vi "Settings Dialog.vi"(8 "error in (no error)":errorcluster, 11 "Settings in":T5={"Acquisition Settings"={"AI"={"task name"="", "task_ref"="", "physical channels"="Dev1/ai0:7", "channels config"={"input terminal configuration"=0, "minimum value"=-5.0, "maximum value"=5.0}, "rate"=1000.0}, "conversions"={"ai0"={"a"=0.0, "b"=0.0}, "ai1"={"a"=0.0, "b"=0.0}, "ai2"={"a"=0.0, "b"=0.0}, "ai3"={"a"=0.0, "b"=0.0}, "ai4"={"a"=0.0, "b"=0.0}}, "compteur 0"={"task name"="CTR", "task_ref"="", "ctr"="Dev1/ctr0:3", "coeff"=4000.0}, "compteur 1"={"task name"="CTR1", "task_ref"="", "ctr"="Dev1/ctr1", "coeff"=4000.0}, "compteur 2"={"task name"="CTR2", "task_ref"="", "ctr"="Dev1/ctr2", "coeff"=4000.0}, "compteur 3"={"task name"="CTR3", "task_ref"="", "ctr"="Dev1/ctr3", "coeff"=4000.0}}, "Logging Configuration"={"Log File Base Path"=path "", "L1"={"ref"=refnum, "actif?"=FALSE, "Fsave"=0.0}, "L2"={"ref"=refnum, "actif?"=FALSE, "Fsave"=0.0}, "L3"={"ref"=refnum, "actif?"=FALSE, "Fsave"=0.0}, "L4"={"ref"=refnum, "actif?"=FALSE, "Fsave"=0.0}}, "Generation Settings"={"AO"={"task name"="AO", "task_ref"="", "physical channels"="Dev1/ao0"}, "PID"={"P"=0.0, "I"=0.0, "D"=0.0}, "conversions"={"ao0"={"a"=0.0, "b"=0.0}}, "setpoint"=0.0}, "Digital Control Configuration"={"DO"={"task name"="DO", "task_ref"="", "lines"="Dev1/port0/line2:3, Dev1/port0/line5"}}} {"Acquisition Settings"."compteur 3"."coeff" format="%0.2f"; "Acquisition Settings"."compteur 2"."coeff" format="%0.2f"; "Acquisition Settings"."compteur 1"."coeff" format="%0.2f"; "Acquisition Settings"."compteur 0"."coeff" format="%0.2f"; "Acquisition Settings"."AI"."rate" format="%0.2f"; "Acquisition Settings"."AI"."channels config"."input terminal configuration" items=["Default"=-1, "RSE"=10083, "NRSE"=10078, "Differential"=10106, "Pseudodifferential"=12529]}) -> (0 "error out":errorcluster, 1 "Cancelled?":bool, 2 "UI Refresh Needed?":bool, 3 "Settings out":T5={"Acquisition Settings"={"AI"={"task name"="", "task_ref"="", "physical channels"="Dev1/ai0:7", "channels config"={"input terminal configuration"=0, "minimum value"=-5.0, "maximum value"=5.0}, "rate"=1000.0}, "conversions"={"ai0"={"a"=0.0, "b"=0.0}, "ai1"={"a"=0.0, "b"=0.0}, "ai2"={"a"=0.0, "b"=0.0}, "ai3"={"a"=0.0, "b"=0.0}, "ai4"={"a"=0.0, "b"=0.0}}, "compteur 0"={"task name"="CTR", "task_ref"="", "ctr"="Dev1/ctr0:3", "coeff"=4000.0}, "compteur 1"={"task name"="CTR1", "task_ref"="", "ctr"="Dev1/ctr1", "coeff"=4000.0}, "compteur 2"={"task name"="CTR2", "task_ref"="", "ctr"="Dev1/ctr2", "coeff"=4000.0}, "compteur 3"={"task name"="CTR3", "task_ref"="", "ctr"="Dev1/ctr3", "coeff"=4000.0}}, "Logging Configuration"={"Log File Base Path"=path "", "L1"={"ref"=refnum, "actif?"=FALSE, "Fsave"=0.0}, "L2"={"ref"=refnum, "actif?"=FALSE, "Fsave"=0.0}, "L3"={"ref"=refnum, "actif?"=FALSE, "Fsave"=0.0}, "L4"={"ref"=refnum, "actif?"=FALSE, "Fsave"=0.0}}, "Generation Settings"={"AO"={"task name"="AO", "task_ref"="", "physical channels"="Dev1/ao0"}, "PID"={"P"=0.0, "I"=0.0, "D"=0.0}, "conversions"={"ao0"={"a"=0.0, "b"=0.0}}, "setpoint"=0.0}, "Digital Control Configuration"={"DO"={"task name"="DO", "task_ref"="", "lines"="Dev1/port0/line2:3, Dev1/port0/line5"}}} {"Acquisition Settings"."compteur 3"."coeff" format="%0.2f"; "Acquisition Settings"."compteur 2"."coeff" format="%0.2f"; "Acquisition Settings"."compteur 1"."coeff" format="%0.2f"; "Acquisition Settings"."compteur 0"."coeff" format="%0.2f"; "Acquisition Settings"."AI"."rate" format="%0.2f"; "Acquisition Settings"."AI"."channels config"."input terminal configuration" items=["Default"=-1, "RSE"=10083, "NRSE"=10078, "Differential"=10106, "Pseudodifferential"=12529]})   [LabVIEW 2014, in "PLS Settings.lvlib"]
doc: "Dialog for selecting user specified settings."
uses:
  PLS Settings.lvlib
  Settings.ctl
  Acquisition/Hardware Configuration.ctl
  conversion.ctl
  Logging/Logging Configuration.ctl
  Generation/Hardware Configuration.ctl
  Digital Control/Hardware Configuration.ctl
  <vilib>/Utility/xml.llb/Write to XML File(string).vi
  Acquisition/PLS Acquisition.lvlib
  Logging/PLS Logging.lvlib
  Generation/PLS Generation.lvlib
  Digital Control/PLS Digital Control.lvlib
panel:
  in  "Digital Control Configuration":T1={"DO"={"task name"="DO", "task_ref"="", "lines"="Dev1/port0/line2:3, Dev1/port0/line5"}}
  in  "reinit":bool
  in  "Generation Settings":T2={"AO"={"task name"="AO", "task_ref"="", "physical channels"="Dev1/ao0"}, "PID"={"P"=0.0, "I"=0.0, "D"=0.0}, "conversions"={"ao0"={"a"=1.0, "b"=0.0}}, "setpoint"=20.0}
  in  "Acquisition Settings":T4={"AI"={"task name"="AI", "task_ref"="", "physical channels"="Dev1/ai3:0, Dev1/ai4", "channels config"={"input terminal configuration"=10083, "minimum value"=0.0, "maximum value"=10.0}, "rate"=10000.0}, "conversions"={"ai0"={"a"=6.725, "b"=-6.25}, "ai1"={"a"=2.69, "b"=-2.5}, "ai2"={"a"=2.69, "b"=-2.5}, "ai3"={"a"=2.69, "b"=-2.5}, "ai4"={"a"=15.0, "b"=0.0}}, "compteur 0"={"task name"="CTR", "task_ref"="", "ctr"="Dev1/ctr0", "coeff"=0.02724}, "compteur 1"={"task name"="CTR1", "task_ref"="", "ctr"="Dev1/ctr1", "coeff"=0.02724}, "compteur 2"={"task name"="CTR2", "task_ref"="", "ctr"="Dev1/ctr2", "coeff"=0.02724}, "compteur 3"={"task name"="CTR3", "task_ref"="", "ctr"="Dev1/ctr3", "coeff"=0.02724}} {"compteur 3"."coeff" format="%#.6f"; "compteur 2"."coeff" format="%#.6f"; "compteur 1"."coeff" format="%#.6f"; "compteur 0"."coeff" format="%#.6f"; "AI"."rate" min=10.0 max=10000.0 step=1.0 format="%d Hz"; "AI"."channels config"."maximum value" min=5.0 max=30.0 step=1.0 format="%d V"; "AI"."channels config"."minimum value" min=-30.0 max=0.0 step=1.0 format="%d V"; "AI"."channels config"."input terminal configuration" items=["Default"=-1, "RSE"=10083, "NRSE"=10078, "Differential"=10106, "Pseudodifferential"=12529]}
  in  "Dossier de résultats":path=path "C:/Users/Public/Documents"
  in  "Cancel Button":bool
  in  "OK Button":bool
  # "Non visible portion of dialog (needed for connector pane)."
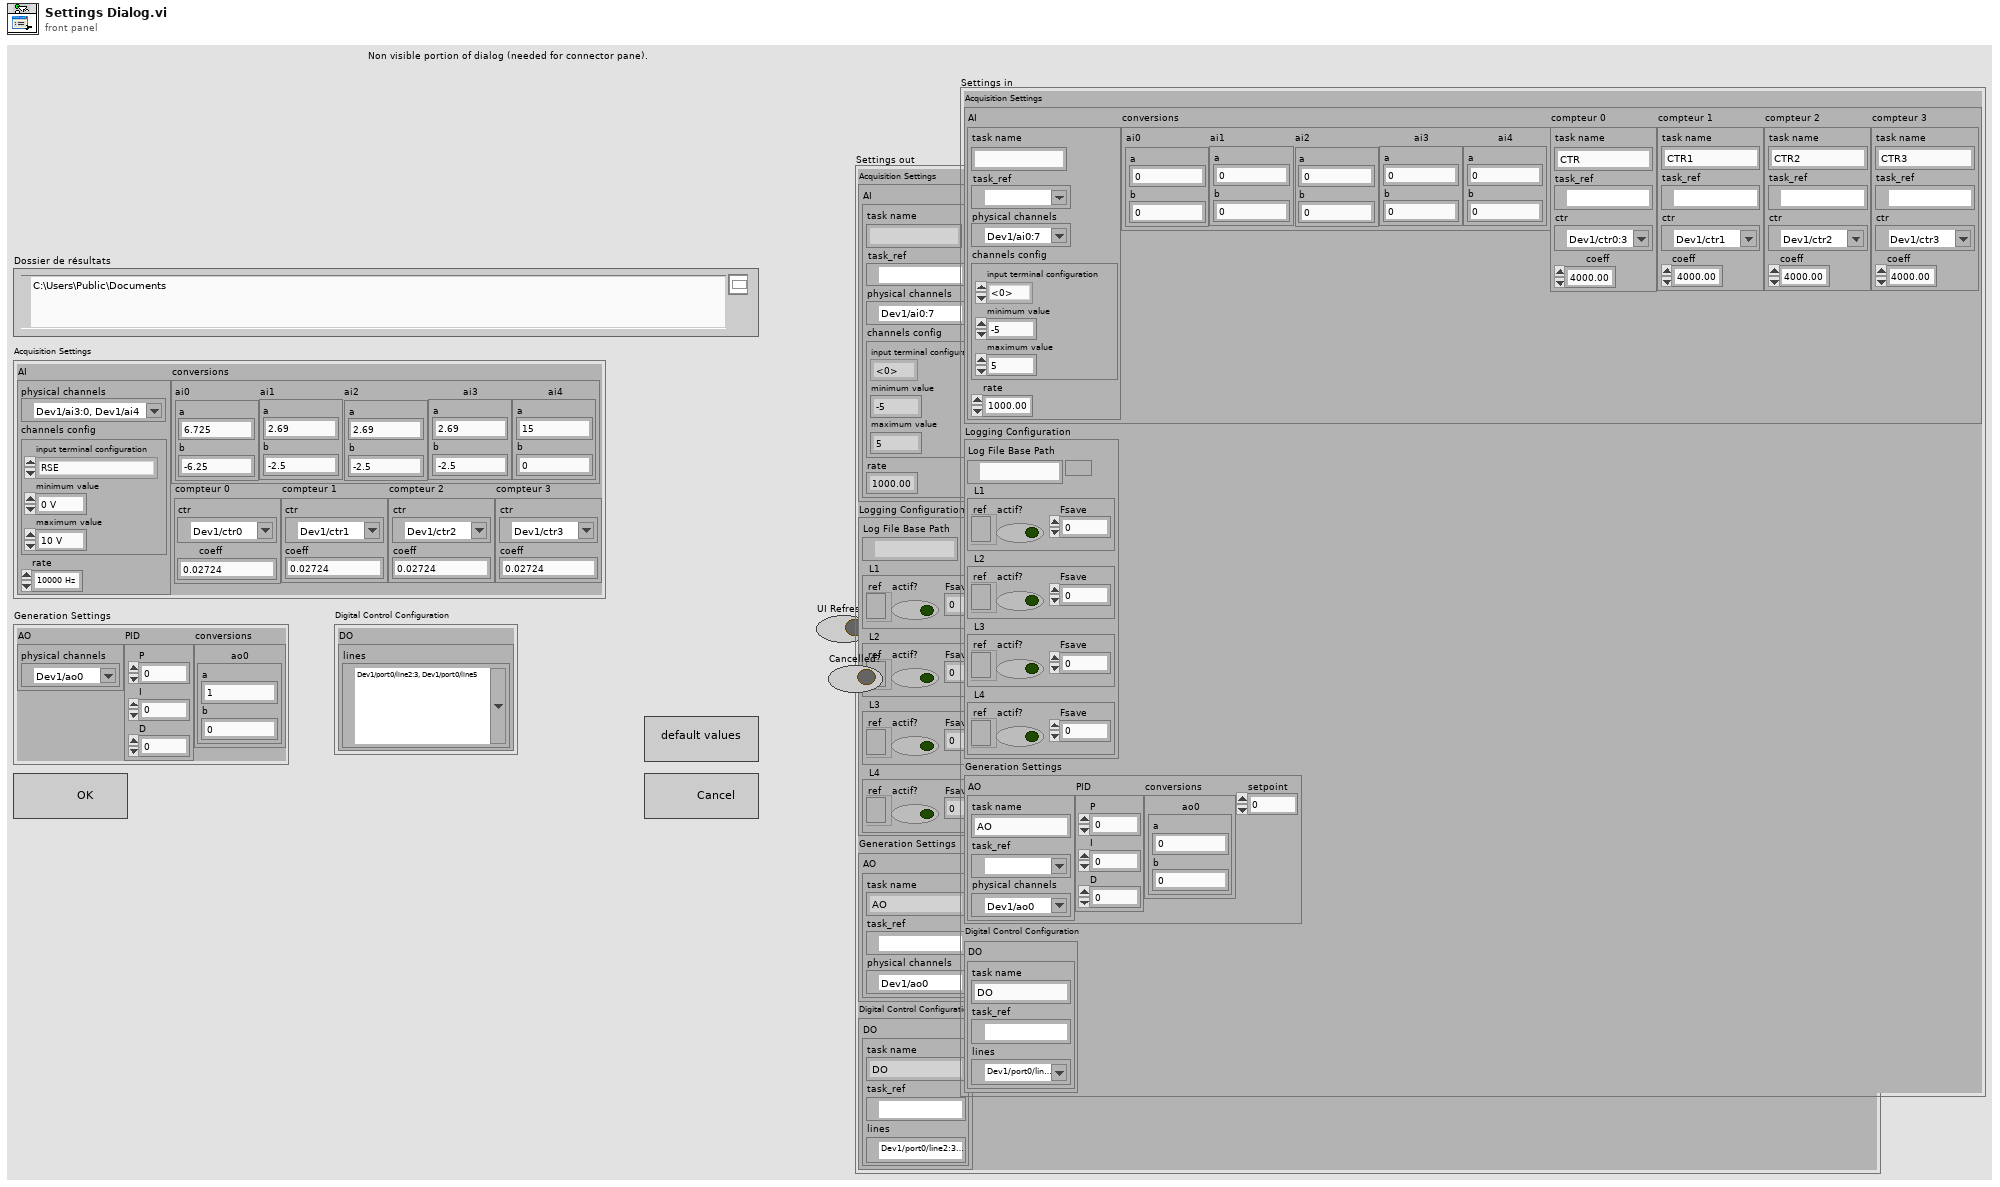
[diagram p1: front panel]
types:
  T1 = typedef "PLS Digital Control.lvlib/Hardware Configuration.ctl" = cluster{"DO":cluster{"task name":string, "task_ref":refnum<k21>, "lines":tag}}
  T2 = typedef "PLS Generation.lvlib/Hardware Configuration.ctl" = cluster{"AO":cluster{"task name":string, "task_ref":refnum<k21>, "physical channels":tag}, "PID":cluster{"P":dbl, "I":dbl, "D":dbl}, "conversions":cluster{"ao0":T3}, "setpoint":dbl}
  T3 = typedef "PLS Settings.lvlib/conversion.ctl" = cluster{"a":dbl, "b":dbl}
  T4 = typedef "PLS Acquisition.lvlib/Hardware Configuration.ctl" = cluster{"AI":cluster{"task name":string, "task_ref":refnum<k21>, "physical channels":tag, "channels config":cluster{"input terminal configuration":i32, "minimum value":dbl, "maximum value":dbl}, "rate":dbl}, "conversions":cluster{"ai0":T3, "ai1":T3, "ai2":T3, "ai3":T3, "ai4":T3}, "compteur 0":cluster{"task name":string, "task_ref":refnum<k21>, "ctr":tag, "coeff":dbl}, "compteur 1":cluster{"task name":string, "task_ref":refnum<k21>, "ctr":tag, "coeff":dbl}, "compteur 2":cluster{"task name":string, "task_ref":refnum<k21>, "ctr":tag, "coeff":dbl}, "compteur 3":cluster{"task name":string, "task_ref":refnum<k21>, "ctr":tag, "coeff":dbl}}
  T5 = typedef "PLS Settings.lvlib/Settings.ctl" = cluster{"Acquisition Settings":T4, "Logging Configuration":T6, "Generation Settings":T2, "Digital Control Configuration":T1}
  T6 = typedef "PLS Logging.lvlib/Logging Configuration.ctl" = cluster{"Log File Base Path":path, "L1":cluster{"ref":refnum<file>, "actif?":bool, "Fsave":dbl}, "L2":cluster{"ref":refnum<file>, "actif?":bool, "Fsave":dbl}, "L3":cluster{"ref":refnum<file>, "actif?":bool, "Fsave":dbl}, "L4":cluster{"ref":refnum<file>, "actif?":bool, "Fsave":dbl}}
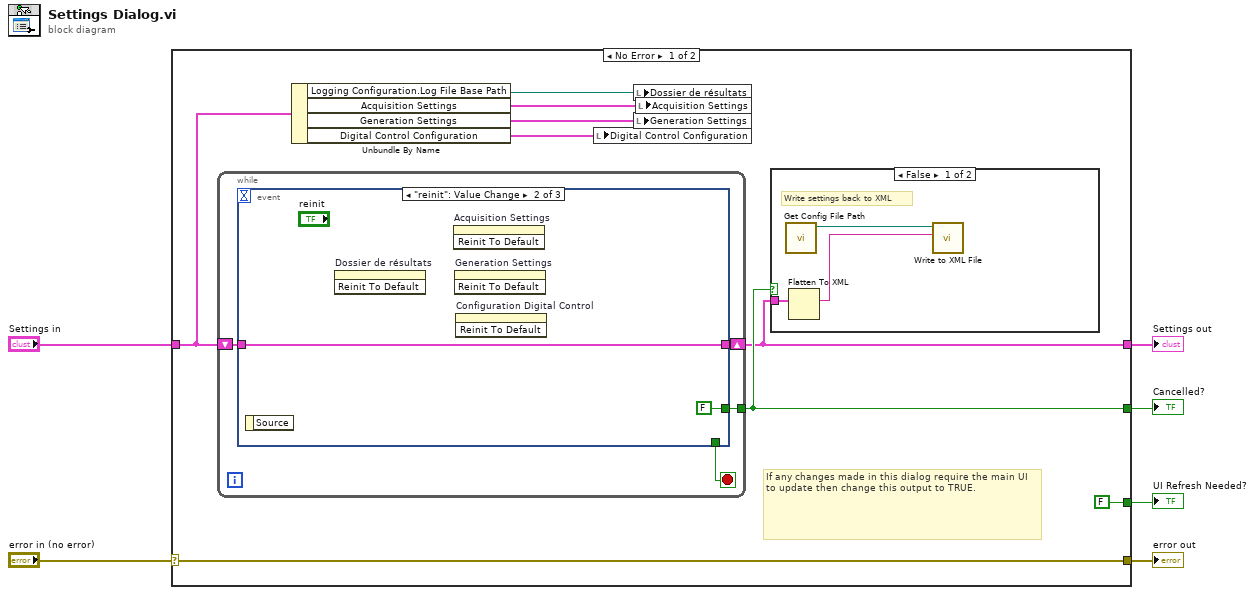
[diagram p0: block diagram]
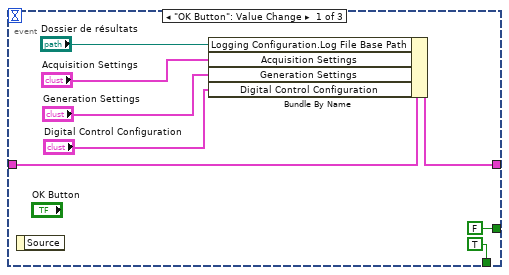
[diagram p2: hidden frame]
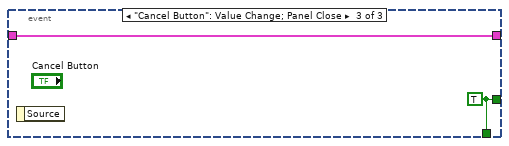
[diagram p3: hidden frame]
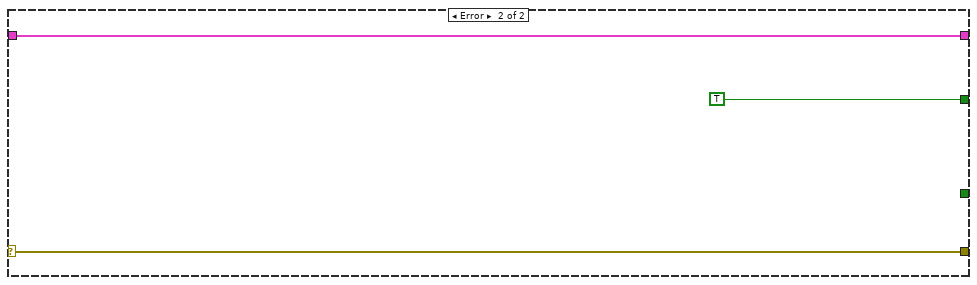
[diagram p5: hidden frame]
diagram:
  n1 = case shown="No Error" "error in (no error)" {
    selector: "error in (no error)" -> [w15 w37]
    tunnel: [w15 w37] -> w5
    tunnel: "Settings in" -> [w11 w36]
    tunnel: [w12 w36] -> w3
    tunnel: [FALSE ("UI Refresh Needed?") _] -> w2
    tunnel: [w13 TRUE ("UI Refresh Needed?")] -> w1
    frame No Error {
      # "If any changes made in this dialog require the main UI to update then change this output to TRUE."
      n2 = while {
        tunnel: [w19] -> w13
        shift-right: [w18] -> w12
        shift-left: w11 -> [w17]
        stop <- w16 stop-if-true
        n3 = event shown="[1] \"reinit\": Value Change" {
          selector: _ -> [_ _ _]
          dyn-events: _ -> [_ _ _]
          timeout: _ -> [_ _ _]
          tunnel: [w26 w28 w31] -> w18
          tunnel: w17 -> [w27 w28 w31]
          tunnel: [FALSE ("UI Refresh Needed?") FALSE ("UI Refresh Needed?") w30] -> w19
          tunnel: [TRUE ("UI Refresh Needed?") _ w30] -> w16
          event "OK Button": Value Change {
            n4 = event-data() -> ()  [unwired: 1 in, 1 out]
            n5 = Bundle By Name(cluster=w27, "Logging Configuration.Log File Base Path"="Dossier de résultats", "Acquisition Settings"="Acquisition Settings", "Generation Settings"="Generation Settings", "Digital Control Configuration"="Digital Control Configuration") -> (w26:T5)
          }
          event "reinit": Value Change {
            n6 = event-data() -> ()  [unwired: 1 in, 1 out]
            n7 = invoke on="Dossier de résultats" class="Path" method="Reinit To Default"() -> ()  [unwired: 3 in, 3 out]
            n8 = invoke on="Acquisition Settings" class="Clust (strict)" method="Reinit To Default"() -> ()  [unwired: 3 in, 3 out]
            n9 = invoke on="Generation Settings" class="Clust (strict)" method="Reinit To Default"() -> ()  [unwired: 3 in, 3 out]
            n10 = invoke on="Configuration Digital Control" class="Clust (strict)" method="Reinit To Default"() -> ()  [unwired: 3 in, 3 out]
          }
          event "Cancel Button": Value Change; Panel Close {
            w30 = TRUE ("UI Refresh Needed?")
            n11 = event-data() -> ()  [unwired: 1 in, 1 out]
          }
        }
      }
      n12 = Unbundle By Name(w11) -> ("Logging Configuration.Log File Base Path"=w10:path, "Acquisition Settings"=w9:T4, "Generation Settings"=w8:T2, "Digital Control Configuration"=w7:T1)
      n13 = local write "Digital Control Configuration"(w7) -> ()
      n14 = local write "Dossier de résultats"(w10) -> ()
      n15 = local write "Generation Settings"(w8) -> ()
      n16 = local write "Acquisition Settings"(w9) -> ()
      n17 = case shown="False" w13 {
        tunnel: w12 -> [w33 _]
        frame False {
          # "Write settings back to XML"
          n18 = call "Get Config File Path.vi"() -> ("XML File Path"=w34:path)  [unwired: 10 in, 1 out]
          n19 = Flatten To XML(anything=w33) -> (xml string=w32:string)
          n20 = call-poly <vilib>:"Write to XML File.vi"("XML Input"=w32, "XML File Path"=w34) -> ()  [unwired: 7 in, 3 out]
        }
        frame True {
        }
      }
    }
    frame Error {
    }
  }
  "UI Refresh Needed?" <- w2
  "error out" <- w5
  "Settings out" <- w3
  "Cancelled?" <- w1
